vi "Read FIFO (Multi-Channel).vi"(2 "FIFO 0":refnum<k21>, 3 "FIFO 1":refnum<k21>, 5 "enabled":bool[](array[boolean])=[FALSE, FALSE], 12 "ready for output":bool) -> (4 "data out":T1[](array[typedef]), 10 "output valid":bool)   [LabVIEW 2023]
doc: "Controls whether or not data is written to the DMA FIFO for the acquisition stream. If burst size is 0, this will be a continuous stream, started when the start trigger is asserted. If burst size is greater than zero, acquisition will be in bursts of the designated size, initiated each time the internal state machine is idle and a start trigger is received.\n\nThis VI also keeps track of whether or not an overflow occurred in the acquisition stream and counts the number of overflows that have occurred for debugging information.\n\nThe internal state machine returns the number of samples processed since the most recent acquisition began and the current state machine state."
uses:
  <instrlib>/_niInstr/Basic Elements/v1/FPGA/Private/Read U32 FIFO.vi
  <instrlib>/_niInstr/DSP/v1/Shared/Public/IQ Data.ctl
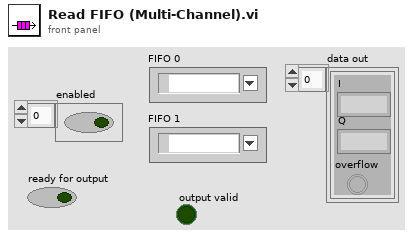
[diagram p1: front panel]
types:
  T1 = typedef "niInstr DSP v1 Shared.lvlib/IQ Data.ctl" = cluster{"I":fxp<+/-,18,1>, "Q":fxp<+/-,18,1>, "overflow":bool}
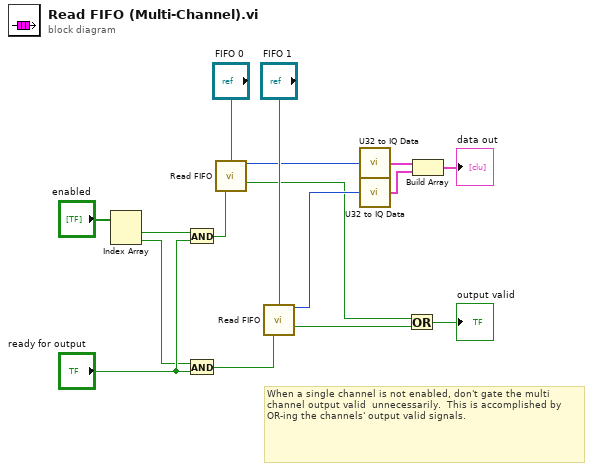
[diagram p0: block diagram]
diagram:
  # "When a single channel is not enabled, don't gate the multi channel output valid  unnecessarily.  This is accomplished by OR-ing the channels' output valid signals."
  n1 = Index Array(array="enabled") -> (element #1=w16:bool, element #2=w1:bool)  [unwired: 2 in]
  n2 = And(x=w16, y="ready for output") -> (x .and. y?=w11:bool)
  n3 = And(x=w1, y="ready for output") -> (x .and. y?=w9:bool)
  n4 = call-poly <instrlib>:"Read FIFO.vi"("fifo"="FIFO 0", "ready for output"=w11) -> ("output data"=w8:u32, "output valid"=w2:bool)  [unwired: 12 in]
  n5 = call-poly <instrlib>:"Read FIFO.vi"("fifo"="FIFO 1", "ready for output"=w9) -> ("output data"=w7:u32, "output valid"=w3:bool)  [unwired: 12 in]
  n6 = call <instrlib>:"U32 to IQ Data.vi"("U32 data"=w8) -> ("IQ data"=w6:T1)  [unwired: 14 in]
  n7 = call <instrlib>:"U32 to IQ Data.vi"("U32 data"=w7) -> ("IQ data"=w5:T1)  [unwired: 14 in]
  n8 = Or(x=w2, y=w3) -> (x .or. y?=→"output valid":bool)
  n9 = Build Array(w6, w5) -> (→"data out":T1[])
